vi "lib_QMH_Set Show Diagram on Init.vi"(8 "error in (no error)":errorcluster caption="错误输入（无错误）", 10 "Show Diagram on Init":bool, 11 "Module Admin in":refnum<class "lib_QMH_Module_Admin.lvclass">) -> (0 "error out":errorcluster caption="错误输出", 3 "Module Admin out":refnum<class "lib_QMH_Module_Admin.lvclass">)   [LabVIEW 2018, in "lib_QMH_Module_Admin.lvclass"]
uses:
  lib_QMH_Module_Admin.lvclass
  lib_QMH_Module_Admin.lvclass/lib_QMH_Module_Admin.ctl
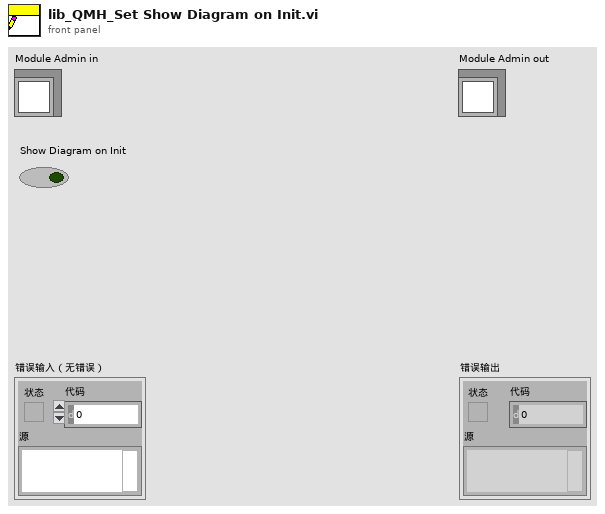
[diagram p1: front panel]
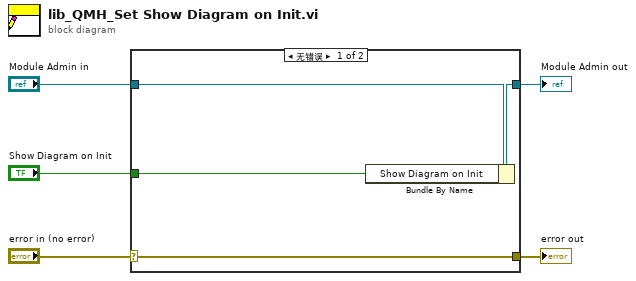
[diagram p0: block diagram]
diagram:
  n1 = case shown="无错误" "error in (no error)" {
    selector: "error in (no error)" -> [w9 w10]
    tunnel: [w9 w10] -> w4
    tunnel: [w7 w11] -> w2
    tunnel: "Module Admin in" -> [w8 w11]
    tunnel: "Show Diagram on Init" -> [w6 _]
    frame No Error {
      n2 = Bundle By Name(cluster=w8, "Show Diagram on Init"=w6) -> (w7:refnum<class "lib_QMH_Module_Admin.lvclass">)
    }
    frame Error {
    }
  }
  "error out" <- w4
  "Module Admin out" <- w2
